vi "DilutionWalker.vi"() -> ()   [LabVIEW 2021]
uses:
  <userlib>/Nanonis Prog Interface V5/Nanonis Prog Interface.lvlib
panel:
  in  "Lockin offset (V)":dbl=0.03
  out "End":bool
  out "Pause":bool
  out "STM RX Temp":dbl
  in  "STM RX\nTemperature Limit (K)":dbl=7.0
  out "Mix Chamber Temp":dbl
  in  "Wait time (ms)":i32=3000
  in  "X Cap Upper limit (mV)":dbl=0.31
  in  "Current limit (nA)":dbl=10.0
  in  "X Cap Lower limit (mV)":dbl=0.22
  in  "Mixing Chamber\nTemperature Limit (K)":dbl=0.7
  in  "?":bool=TRUE
  in  "Number of Steps Increment":i32=200
  out "Z capacitance (pA)":cluster{"y":i32, sgl}[](graph)
  out "X capacitance (mV)":cluster{"y":i32, dbl}[](graph)
  in  "Lockin sensitivity (V)":dbl=0.02
  out "X capacitance (mV)":sgl
  out "Current (pA)":sgl
  out "Z capacitance (pA)":sgl
  # "+X"
  # "-X"
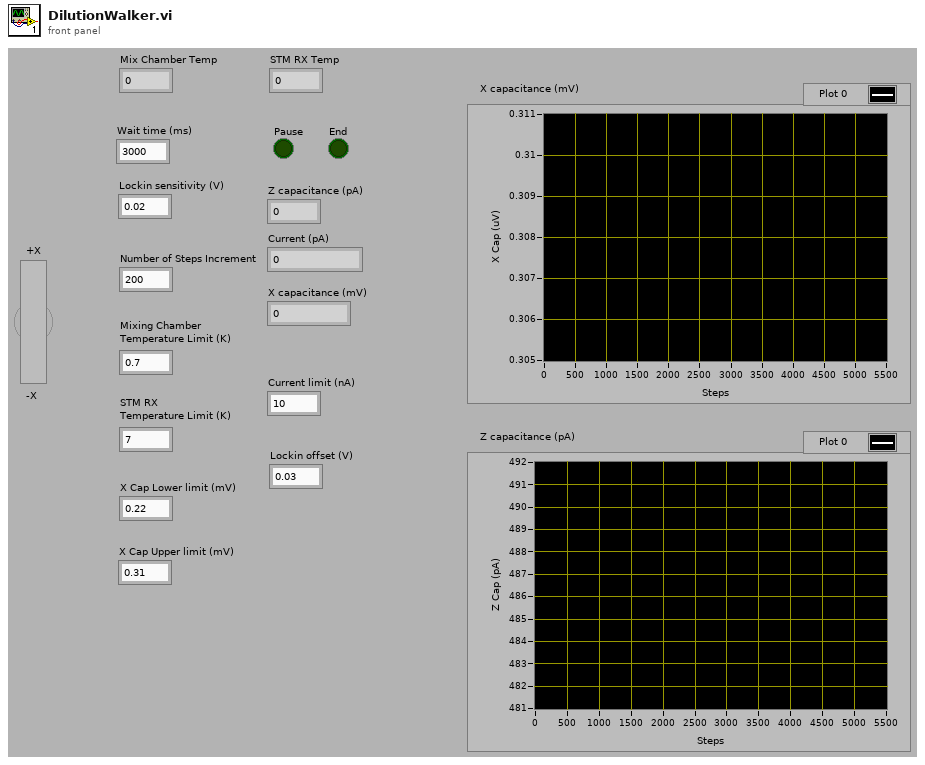
[diagram p1: front panel]
types:
  T1 = enum16{"Set Heater Voltage", "Read Heater Voltage", "Read Heater Current", "Read 1K Pot Temperature", "Read IVC Sorb Temperature", "Read Needle Valve Temperature", "Read Still Pressure", "Read Mixing Chamber Temperature", "Read STM RX Temperature", "Read STM CX Temperature", "Unstall Triton Loop", "Triton Stop", "Triton Stall Status"}
  T2 = enum8{"Group 1", "Group 2", "Group 3", "Group 4", "Group 5", "Group 6"}
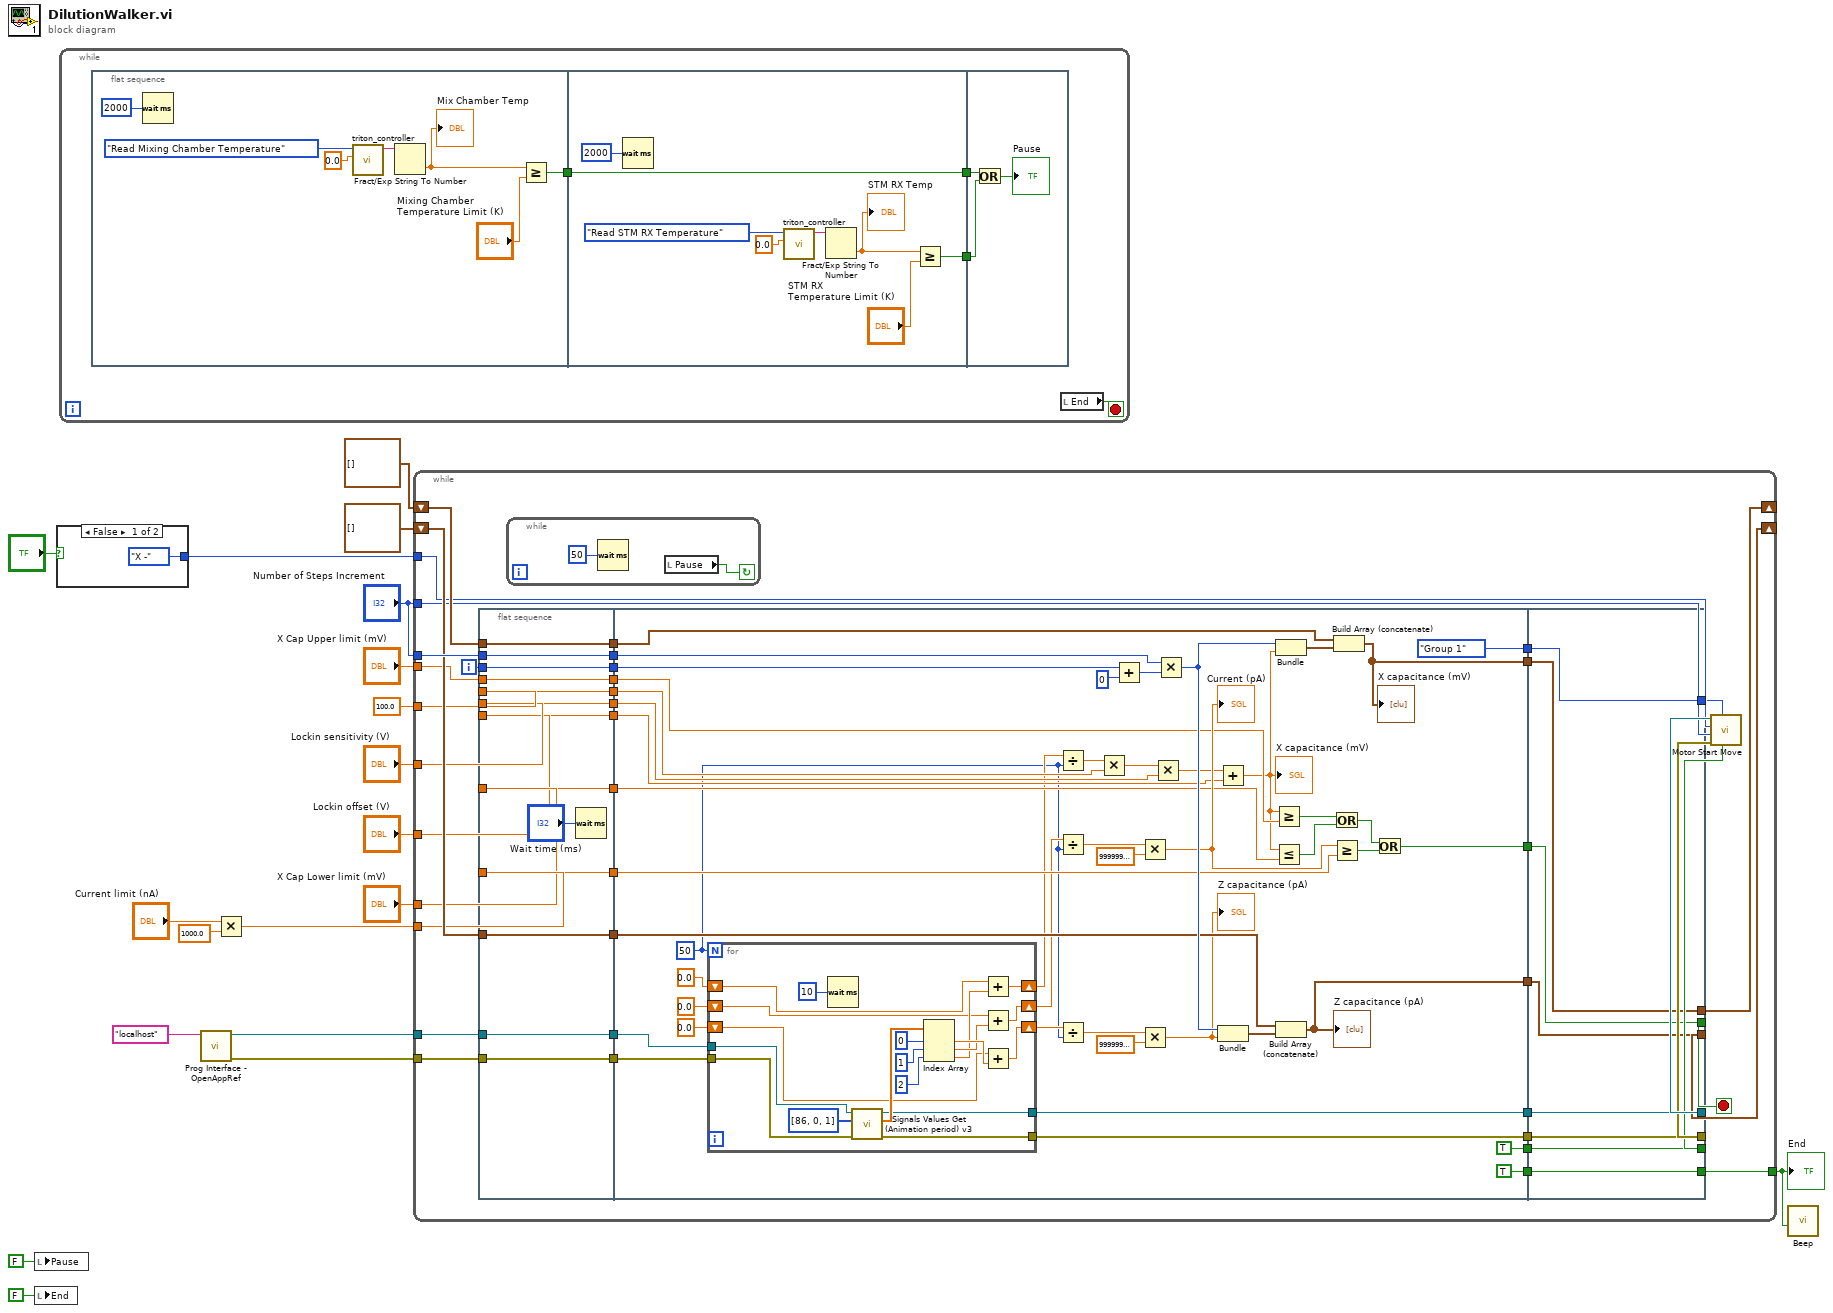
[diagram p0: block diagram]
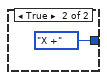
[diagram p2: hidden frame]
diagram:
  n1 = local write "Pause"(FALSE ("Pause")) -> ()
  n2 = local write "End"(FALSE ("End")) -> ()
  n3 = case shown="False" "?" {
    tunnel: [enum16{"X +", "X -", "Y +", "Y -", "Z +", "Z -"}."X -" ("Direction") enum16{"X +", "X -", "Y +", "Y -", "Z +", "Z -"}."X +" ("Direction")] -> w17
    frame False {
    }
    frame True {
    }
  }
  n4 = while {
    stop <- w22 stop-if-true
    n5 = flat-sequence {
      tunnel: [w26] -> w23
      tunnel: [w34] -> w25
      tunnel: [w33] -> w24
      tunnel: w23 -> [w33]
      tunnel: w25 -> [w43]
      tunnel: w24 -> [w42]
      frame #0 {
        n6 = Wait (ms)(milliseconds to wait=u32 2000) -> ()  [unwired: 1 out]
        n7 = call "triton_controller.vi"("Numerical Argument"=0.0, "Command"=T1."Read Mixing Chamber Temperature") -> ("Response"=w29:string)  [unwired: 9 in]
        n8 = Fract/Exp String To Number(string=w29) -> (number=w28:dbl)  [unwired: 3 in, 1 out]
        "Mix Chamber Temp" <- w28
        n9 = Greater Or Equal?(x=w28, y="Mixing Chamber\nTemperature Limit (K)") -> (x >= y?=w26:bool)
      }
      frame #1 {
        n10 = Wait (ms)(milliseconds to wait=u32 2000) -> ()  [unwired: 1 out]
        n11 = call "triton_controller.vi"("Numerical Argument"=0.0, "Command"=T1."Read STM RX Temperature") -> ("Response"=w37:string)  [unwired: 9 in]
        n12 = Fract/Exp String To Number(string=w37) -> (number=w35:dbl)  [unwired: 3 in, 1 out]
        "STM RX Temp" <- w35
        n13 = Greater Or Equal?(x=w35, y="STM RX\nTemperature Limit (K)") -> (x >= y?=w34:bool)
      }
      frame #2 {
        n14 = Or(x=w42, y=w43) -> (x .or. y?=→"Pause":bool)
      }
    }
    n15 = local read "End"() -> (w22:bool)
  }
  n16 = call <userlib>:"Prog Interface - OpenAppRef.vi"("Machine name (local machine IP)"="localhost" ("machine name (localhost)")) -> ("Error out"=w1:errorcluster, "Application reference"=w2:refnum<vi>)  [unwired: 5 in]
  n17 = Multiply(x="Current limit (nA)", y=1000.0) -> (x*y=w11:dbl)
  n18 = while {
    tunnel: w1 -> [w85]
    tunnel: w2 -> [w84]
    tunnel: "Lockin sensitivity (V)" -> [w68]
    tunnel: "Number of Steps Increment" -> [w83]
    shift-right: [w72] -> _
    shift-left: cluster{i32, sgl}[] [] -> [w82]
    shift-right: [w73] -> _
    shift-left: cluster{i32, sgl}[] [] -> [w81]
    tunnel: w17 -> [w77]
    tunnel: "Number of Steps Increment" -> [w76]
    tunnel: [w74] -> w15
    tunnel: 100.0 ("y") -> [w71]
    tunnel: w11 -> [w70]
    tunnel: "X Cap Upper limit (mV)" -> [w67]
    tunnel: "X Cap Lower limit (mV)" -> [w66]
    tunnel: "Lockin offset (V)" -> [w64]
    i -> [w69]
    stop <- w65 stop-if-true
    n19 = flat-sequence {
      tunnel: w64 -> [w87]
      tunnel: w66 -> [w88]
      tunnel: w67 -> [w89]
      tunnel: w68 -> [w90]
      tunnel: w69 -> [w91]
      tunnel: w70 -> [w92]
      tunnel: w71 -> [w93]
      tunnel: w81 -> [w94]
      tunnel: w82 -> [w95]
      tunnel: w83 -> [w96]
      tunnel: w84 -> [w97]
      tunnel: w85 -> [w98]
      tunnel: [w98] -> w55
      tunnel: [w97] -> w54
      tunnel: [w96] -> w53
      tunnel: [w95] -> w52
      tunnel: [w94] -> w51
      tunnel: [w93] -> w50
      tunnel: [w92] -> w49
      tunnel: [w91] -> w48
      tunnel: [w90] -> w47
      tunnel: [w89] -> w46
      tunnel: [w88] -> w45
      tunnel: [w87] -> w44
      tunnel: [w132] -> w63
      tunnel: [w131] -> w62
      tunnel: [TRUE ("Wait until finished? (F)")] -> w61
      tunnel: [T2."Group 1" ("Group")] -> w60
      tunnel: [TRUE] -> w59
      tunnel: [w127] -> w58
      tunnel: [w126] -> w57
      tunnel: [w112] -> w56
      tunnel: w55 -> [w144]
      tunnel: w54 -> [w143]
      tunnel: w53 -> [w138]
      tunnel: w52 -> [w136]
      tunnel: w51 -> [w133]
      tunnel: w50 -> [w125]
      tunnel: w49 -> [w123]
      tunnel: w48 -> [w121]
      tunnel: w47 -> [w120]
      tunnel: w46 -> [w118]
      tunnel: w45 -> [w117]
      tunnel: w44 -> [w109]
      tunnel: [w164] -> w65
      tunnel: [w165] -> w72
      tunnel: [w166] -> w73
      tunnel: [w167] -> w74
      tunnel: [w168] -> w75
      tunnel: [w169] -> w78
      tunnel: [w170] -> w79
      tunnel: [w171] -> w80
      tunnel: w63 -> [w171]
      tunnel: w62 -> [w170]
      tunnel: w61 -> [w169]
      tunnel: w60 -> [w168]
      tunnel: w59 -> [w167]
      tunnel: w58 -> [w166]
      tunnel: w57 -> [w165]
      tunnel: w56 -> [w164]
      frame #0 {
        n20 = Wait (ms)(milliseconds to wait="Wait time (ms)") -> ()  [unwired: 1 out]
      }
      frame #1 {
        w99 = 50
        n21 = for {
          N: w99 -> [_]
          tunnel: w144 -> [w163]
          tunnel: w143 -> [w159]
          tunnel: [w156] -> w132
          tunnel: [w155] -> w131
          shift-right: [w152] -> w104
          shift-left: sgl 0.0 -> [w147]
          shift-right: [w151] -> w100
          shift-left: sgl 0.0 -> [w146]
          shift-right: [w148] -> w102
          shift-left: sgl 0.0 -> [w145]
          n22 = Wait (ms)(milliseconds to wait=u32 10) -> ()  [unwired: 1 out]
          n23 = call <userlib>:"Signals Values Get (Animation period) v3.vi"("error in (no error)"=w163, "Signals indexes (0-127)"=i8[] [86, 0, 1], "Application ref in"=w159) -> ("error out"=w155:errorcluster, "Signals Values"=w161:sgl[], "Application ref out"=w156:refnum<vi>)  [unwired: 5 in]
          n24 = Index Array(array=w161, index #1=0 ("index"), index #2=1 ("index"), index #3=2 ("index")) -> (element #1=w153:sgl, element #2=w150:sgl, element #3=w149:sgl)
          n25 = Add(x=w145, y=w149) -> (x+y=w148:sgl)
          n26 = Add(x=w146, y=w150) -> (x+y=w151:sgl)
          n27 = Add(x=w147, y=w153) -> (x+y=w152:sgl)
        }
        n28 = Divide(x=w102, y=w99) -> (x/y=w103:sgl)
        n29 = Divide(x=w100, y=w99) -> (x/y=w101:sgl)
        n30 = Divide(x=w104, y=w99) -> (x/y=w105:sgl)
        n31 = Multiply(x=w103, y=w125) -> (x*y=w119:dbl)
        n32 = Add(x=w121, y=u16 0) -> (x+y=w139:i32)
        n33 = Multiply(x=w101, y=sgl 1000000000000.0) -> (x*y=w124:sgl)
        "Current (pA)" <- w124
        n34 = Multiply(x=w105, y=sgl 1000000000000.0) -> (x*y=w122:sgl)
        "Z capacitance (pA)" <- w122
        n35 = Multiply(x=w119, y=w120) -> (x*y=w110:dbl)
        n36 = Multiply(x=w138, y=w139) -> (x*y=w135:i32)
        n37 = Add(x=w110, y=w109) -> (x+y=w111:dbl)
        "X capacitance (mV)" <- w111
        n38 = Bundle(w135, w122) -> (w134:cluster{i32, sgl})  [unwired: 1 in]
        n39 = Greater Or Equal?(x=w111, y=w118) -> (x >= y?=w116:bool)
        n40 = Less Or Equal?(x=w111, y=w117) -> (x <= y?=w115:bool)
        n41 = Bundle(w135, w111) -> (w137:cluster{i32, dbl})  [unwired: 1 in]
        n42 = Build Array (concatenate)(w133, w134) -> (w127:cluster{i32, sgl}[])
        "Z capacitance (pA)" <- w127
        n43 = Or(x=w116, y=w115) -> (x .or. y?=w114:bool)
        n44 = Greater Or Equal?(x=w124, y=w123) -> (x >= y?=w113:bool)
        n45 = Build Array (concatenate)(w136, w137) -> (w126:cluster{i32, dbl}[])
        "X capacitance (mV)" <- w126
        n46 = Or(x=w114, y=w113) -> (x .or. y?=w112:bool)
      }
      frame #2 {
      }
    }
    n47 = while {
      stop <- w173 continue-if-true
      n48 = Wait (ms)(milliseconds to wait=u32 50) -> ()  [unwired: 1 out]
      n49 = local read "Pause"() -> (w173:bool)
    }
    n50 = call <userlib>:"Motor Start Move.vi"("Wait until finished? (F)"=w78, "Group"=w75, "Error in (no error)"=w79, "Number of steps"=w76, "Direction"=w77, "Application ref in"=w80) -> ()  [unwired: 3 in, 2 out]
  }
  "End" <- w15
  n51 = call <vilib>:"Beep.vi"("use system alert? (T)"=w15) -> ()  [unwired: 11 in]
